vi "AviPlay.vi"(7 "Numeric Iteration":i32, 8 "error in (no error)":errorcluster, 9 "New Image":T2, 10 "Seconds per Frame":dbl, 11 "Refnum in Avi":T1) -> (0 "error out":errorcluster, 1 "Progress Bar":i32(slide) max=115 scale=1.0..115.0, 2 "Image Out":T2, 3 "Refnum out Avi":T1)   [LabVIEW 2015]
uses:
  <vilib>/vision/Image Controls.llb/IMAQ Image.ctl
  <vilib>/vision/Avi.llb/IMAQ AVI2 Refnum.ctl
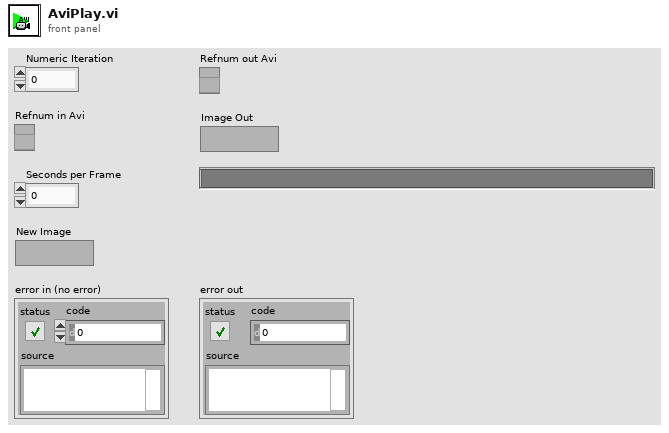
[diagram p1: front panel]
types:
  T1 = typedef "IMAQ AVI2 Refnum.ctl" = refnum<k20>
  T2 = typedef "IMAQ Image.ctl" = refnum<image>
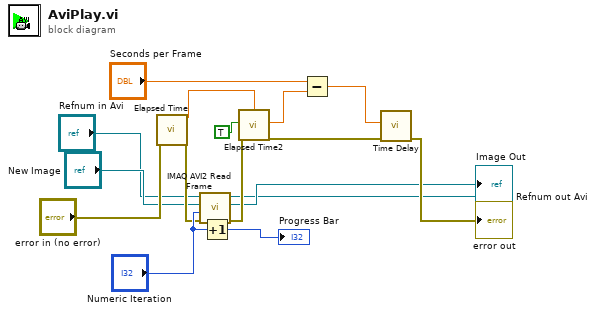
[diagram p0: block diagram]
diagram:
  n1 = call "Elapsed Time"("error in (no error)"="error in (no error)") -> ("Present (s)"=w9:dbl, "error out"=w5:errorcluster)  [unwired: 11 in, 6 out]
  n2 = call "IMAQ AVI2 Read Frame"("error in (no error)"=w5, "Frame Number"="Numeric Iteration", "Image"="New Image", "AVI Refnum"="Refnum in Avi") -> ("error out"=w11:errorcluster, "Image Out"=→"Image Out":T2, "AVI Refnum (duplicate)"=→"Refnum out Avi":T1)  [unwired: 5 out]
  n3 = Increment(x="Numeric Iteration") -> (x+1=→"Progress Bar":i32)
  n4 = call "Elapsed Time2"("Reset"=TRUE, "error in (no error)"=w11, "Set Start Time (s)"=w9) -> ("Elapsed Time (s)"=w12:dbl, "error out"=w13:errorcluster)  [unwired: 9 in, 6 out]
  n5 = Subtract(x="Seconds per Frame", y=w12) -> (x-y=w7:dbl)
  n6 = call "Time Delay"("error in (no error)"=w13, "Delay Time (s)"=w7) -> ("error out"=→"error out":errorcluster)  [unwired: 9 in]
